vi "extractElementBasicType.vi"(8 "error in (no error)":errorcluster, 11 "Topic in":refnum<class "Topic.lvclass">) -> (0 "error out":errorcluster, 2 "elementBasicType":string, 3 "Topic out":refnum<class "Topic.lvclass">)   [LabVIEW 2016, in "Topic.lvclass"]
uses:
  Topic.lvclass
  Topic.lvclass/Topic.ctl
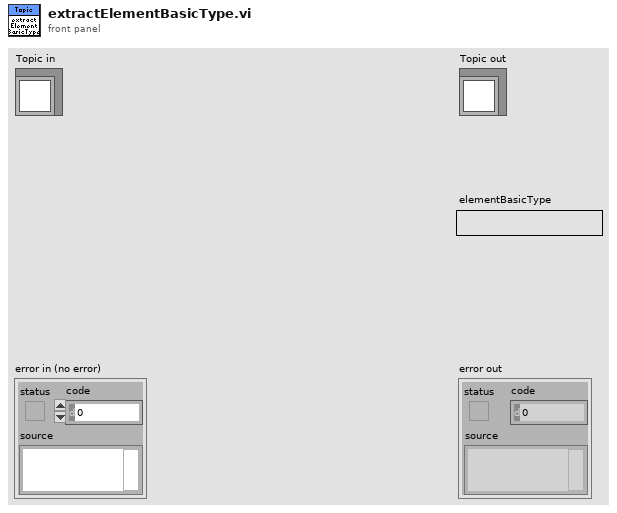
[diagram p1: front panel]
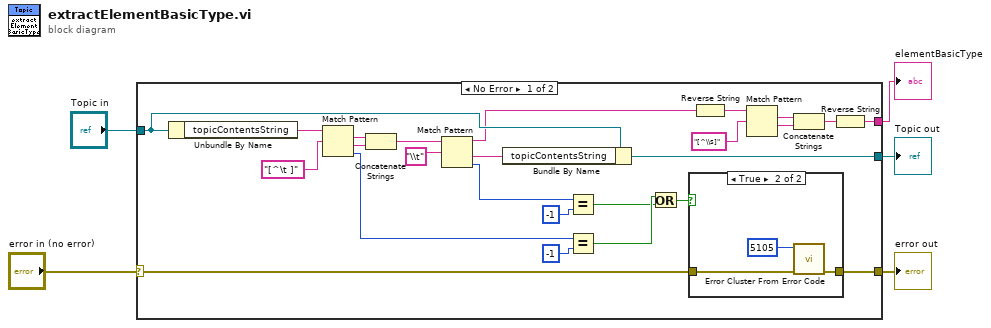
[diagram p0: block diagram]
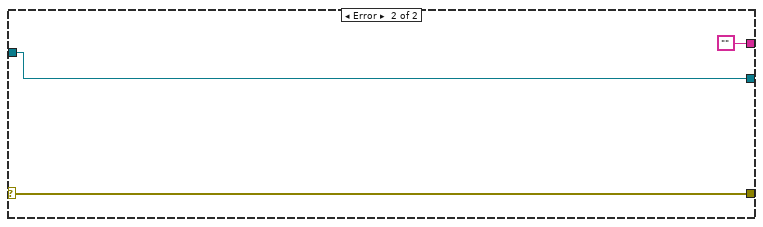
[diagram p3: hidden frame]
diagram:
  n1 = case shown="No Error" "error in (no error)" {
    selector: "error in (no error)" -> [w13 w37]
    tunnel: [w12 w37] -> w4
    tunnel: [w29 w36] -> w2
    tunnel: "Topic in" -> [w30 w36]
    tunnel: [w9 ""] -> w1
    frame No Error {
      n2 = Unbundle By Name(w30) -> ("topicContentsString"=w16:string)
      n3 = Match Pattern(string=w16, regular expression="[^\t ]") -> (match substring=w19:string, after substring=w18:string, offset past match=w27:i32)  [unwired: 1 in, 1 out]
      n4 = Concatenate Strings(w19, w18) -> (w17:string)
      n5 = Match Pattern(string=w17, regular expression="\\t") -> (before substring=w10:string, after substring=w15:string, offset past match=w25:i32)  [unwired: 1 in, 1 out]
      n6 = Bundle By Name(cluster=w30, "topicContentsString"=w15) -> (w29:refnum<class "Topic.lvclass">)
      n7 = Equal?(x=w25, y=-1) -> (x = y?=w22:bool)
      n8 = Equal?(x=w27, y=-1) -> (x = y?=w23:bool)
      n9 = Or(x=w23, y=w22) -> (x .or. y?=w14:bool)
      n10 = case shown="True" w14 {
        tunnel: w13 -> [w31 w33]
        tunnel: [w31 w32] -> w12
        frame False {
        }
        frame True {
          n11 = call <vilib>:"Error Cluster From Error Code.vi"("error in (no error)"=w33, "error code (0)"=5105) -> ("error out"=w32:errorcluster)  [unwired: 7 in]
        }
      }
      n12 = Reverse String(1:w10) -> (0:w11:string)
      n13 = Match Pattern(string=w11, regular expression="[^\\s]") -> (match substring=w8:string, after substring=w7:string)  [unwired: 1 in, 2 out]
      n14 = Concatenate Strings(w8, w7) -> (w6:string)
      n15 = Reverse String(1:w6) -> (0:w9:string)
    }
    frame Error {
    }
  }
  "error out" <- w4
  "Topic out" <- w2
  "elementBasicType" <- w1
